vi "BASE_Setting.vi"(8 "error in (no error)":errorcluster) -> (0 "error out":errorcluster)   [LabVIEW 2017]
doc: "this is Hardware setting to set ip address and com port of scanner"
panel:
  in  "System Tab":enum32{"COMMUNICATION SETTING"}(tab)
  in  "HardwareSetting":T1
  in  "Save Button":bool
  in  "Default Button":bool
  in  "Back":bool
  # "BARCODE VERIFICATION SYSTEM REPORTS"
  # "Hardware Setting"
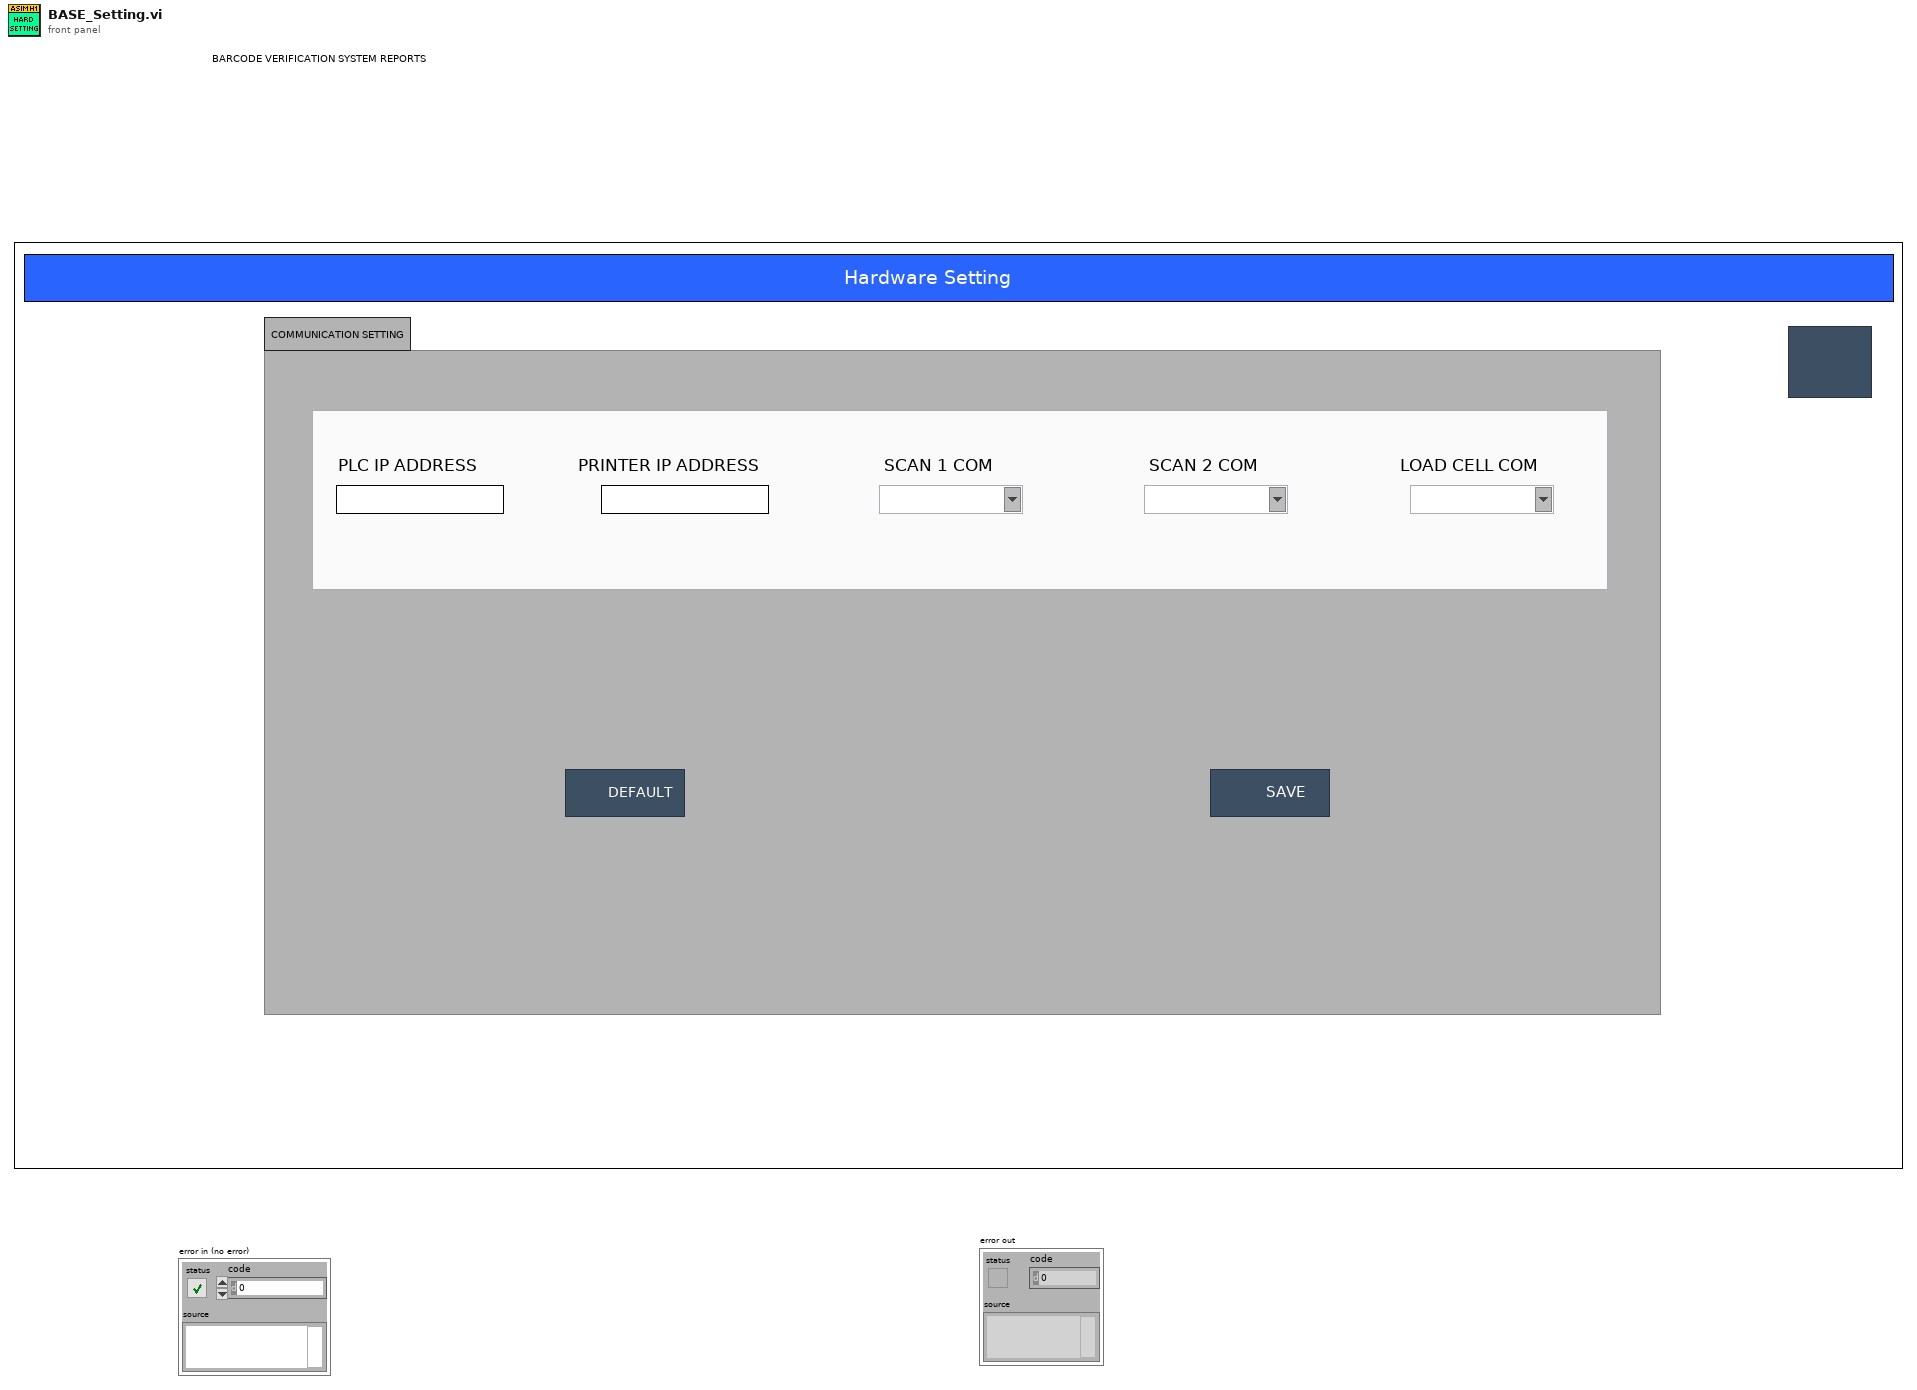
[diagram p1: front panel]
types:
  T1 = cluster{"PLC IP ADDRESS":string, "SCAN 1 COM":refnum<visa-resource-name>, "SCAN 2 COM":refnum<visa-resource-name>, "LOAD CELL COM":refnum<visa-resource-name>, "PRINTER IP ADDRESS":string}
  T2 = enum32{"invalid app kind", "Development System", "Run Time System", "Student Edition", "Embedded LabVIEW", "Evaluation", "Custom"}
  T3 = enum32{"Invalid", "Standard", "Closed", "Hidden", "Minimized", "Maximized"}
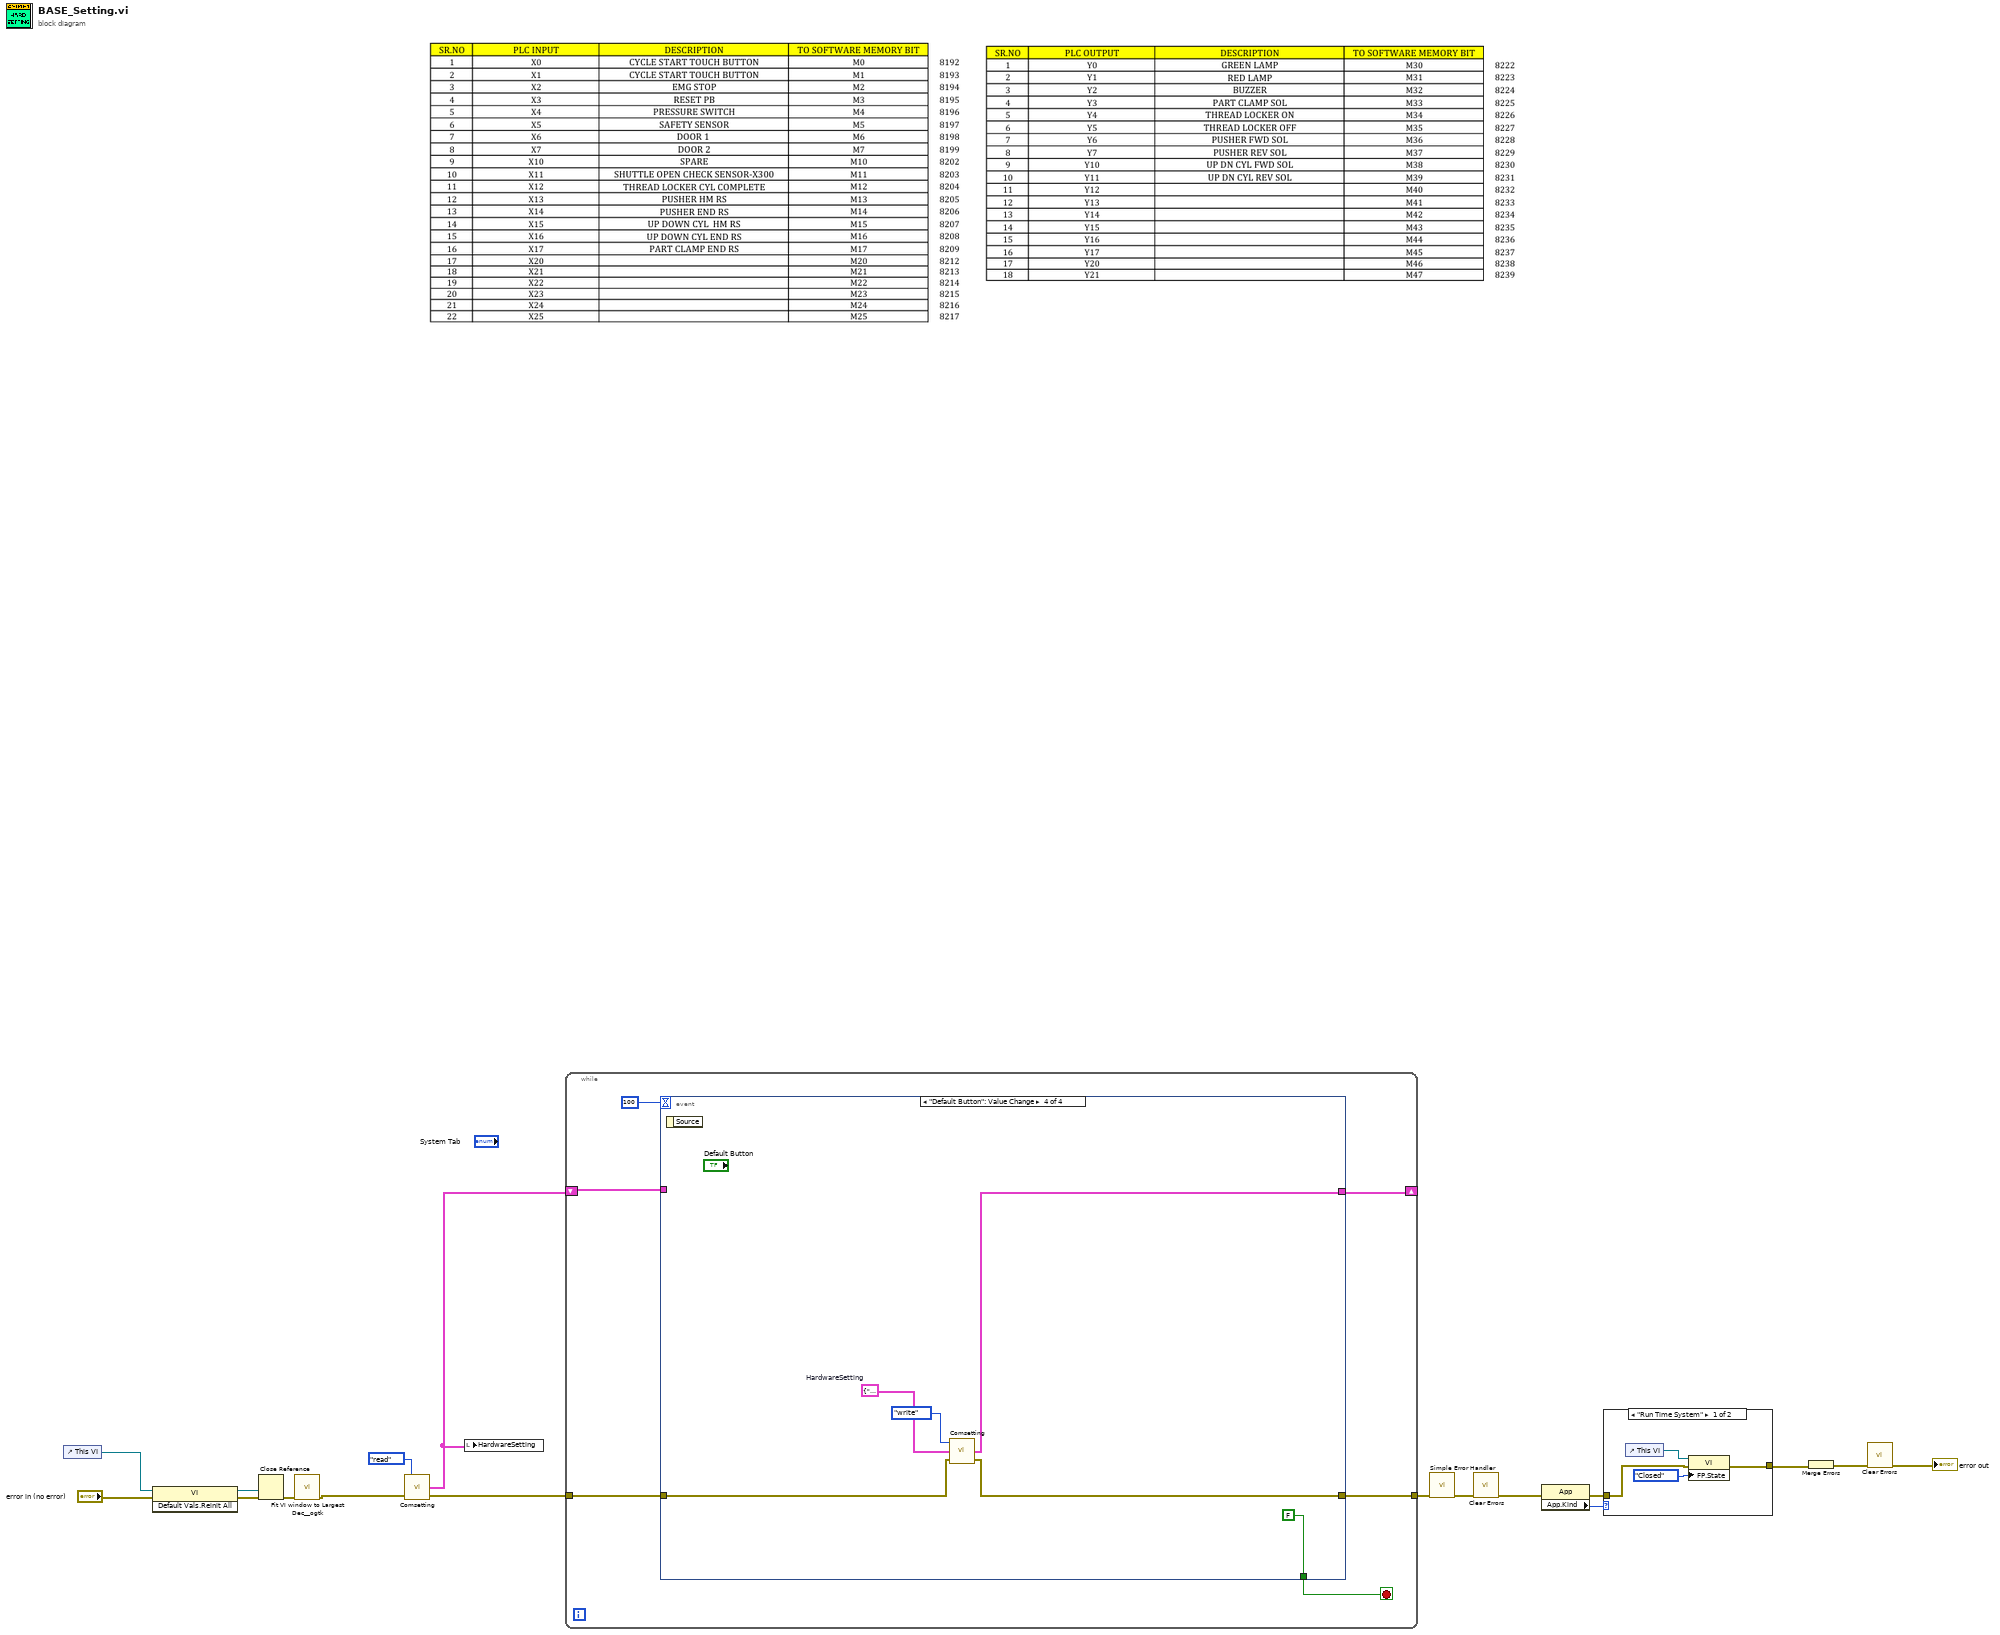
[diagram p0: block diagram]
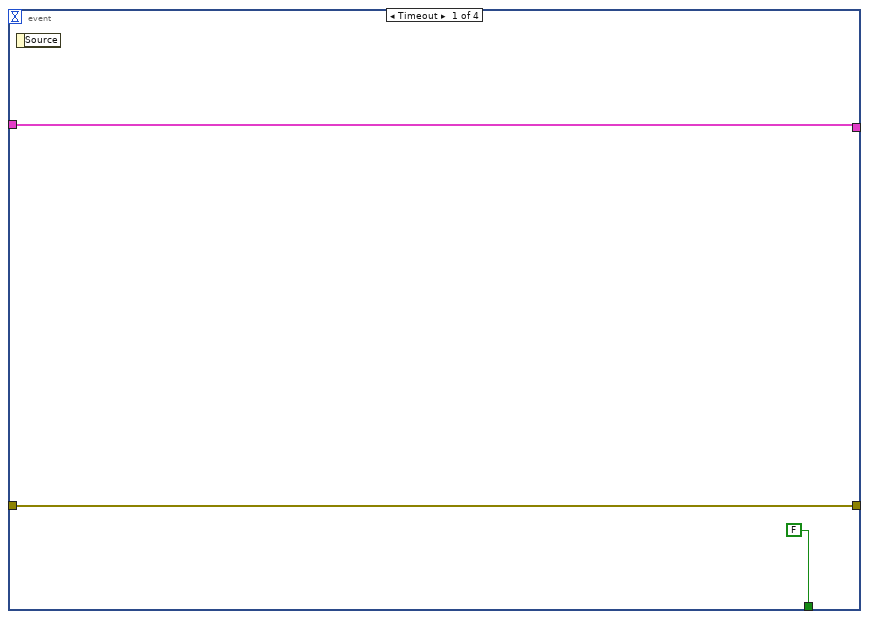
[diagram p2: hidden frame]
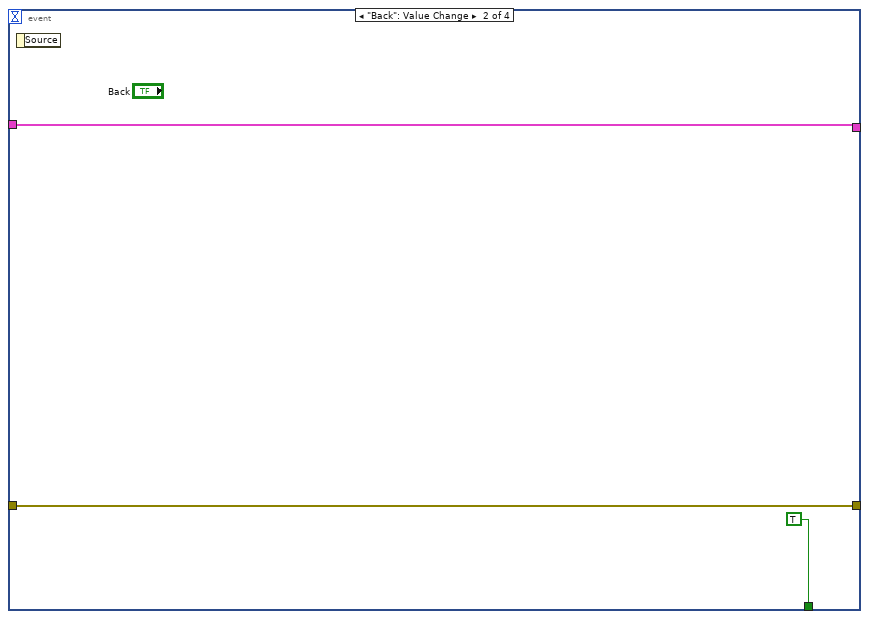
[diagram p3: hidden frame]
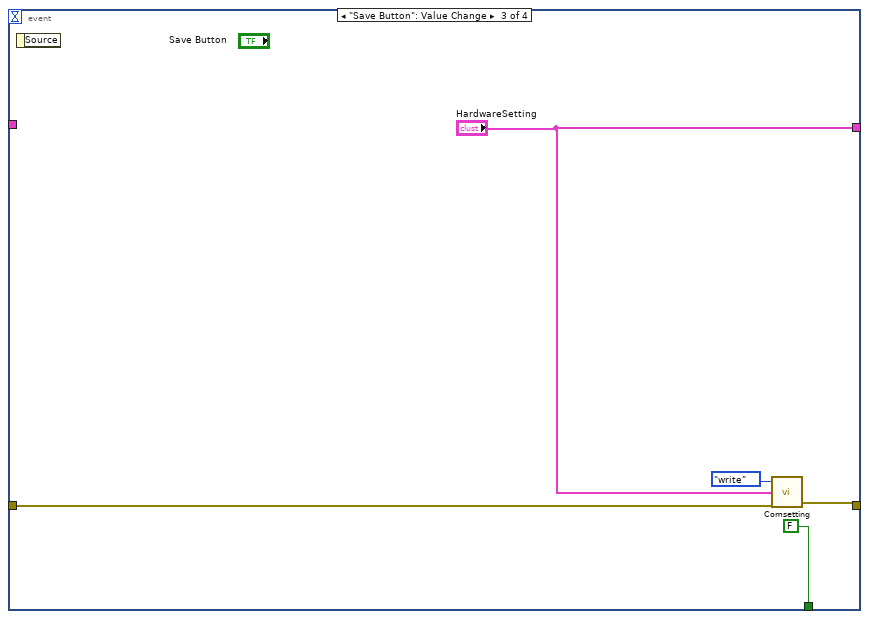
[diagram p4: hidden frame]
diagram:
  n1 = control-ref of="This VI"() -> (w14:refnum<vi>)
  n2 = invoke class="VI" method="Default Vals.Reinit All"(reference=w14, error in="error in (no error)") -> (reference out=w12:refnum<vi>, error out=w11:errorcluster)  [unwired: 1 in, 1 out]
  n3 = Close Reference(reference=w12, error in (no error)=w11) -> (error out=w10:errorcluster)
  n4 = call <userlib>:"Fit VI window to Largest Dec__ogtk.vi"("error in (no error)"=w10) -> ("error out"=w3:errorcluster)  [unwired: 5 in, 1 out]
  n5 = call "Comsetting.vi"("error in"=w3, "Enum"=enum16{"read", "write"}."read") -> ("error our"=w2:errorcluster, "HardwareSetting"=w1:T1)  [unwired: 1 in, 1 out]
  n6 = local write "HardwareSetting"(w1) -> ()
  n7 = while {
    tunnel: [w23] -> w4
    tunnel: w2 -> [w22]
    shift-right: [w21] -> _
    shift-left: w1 -> [w20]
    stop <- w18 stop-if-true
    n8 = event shown="[3] \"Default Button\": Value Change" {
      selector: _ -> [_ _ _ _]
      dyn-events: _ -> [_ _ _ _]
      timeout: 100 -> [_ _ _ _]
      tunnel: [w24 w28 w33 w39] -> w23
      tunnel: w22 -> [w24 w28 w34 w40]
      tunnel: w20 -> [w26 w27 _ _]
      tunnel: [w26 w27 "HardwareSetting" w37] -> w21
      tunnel: [FALSE TRUE FALSE FALSE] -> w18
      event Timeout {
        n9 = event-data() -> ()  [unwired: 1 in, 1 out]
      }
      event "Back": Value Change {
        n10 = event-data() -> ()  [unwired: 1 in, 1 out]
      }
      event "Save Button": Value Change {
        n11 = event-data() -> ()  [unwired: 1 in, 1 out]
        n12 = call "Comsetting.vi"("error in"=w34, "HardwareSetting"="HardwareSetting", "Enum"=enum16{"read", "write"}."write") -> ("error our"=w33:errorcluster)  [unwired: 2 out]
      }
      event "Default Button": Value Change {
        w35 = T1 {"PLC IP ADDRESS"="", "SCAN 1 COM"="", "SCAN 2 COM"="", "LOAD CELL COM"="", "PRINTER IP ADDRESS"=""}  # HardwareSetting
        n13 = event-data() -> ()  [unwired: 1 in, 1 out]
        n14 = call "Comsetting.vi"("error in"=w40, "HardwareSetting"=w35, "Enum"=enum16{"read", "write"}."write") -> ("error our"=w39:errorcluster, "HardwareSetting"=w37:T1)  [unwired: 1 out]
      }
    }
  }
  n15 = call <vilib>:"Simple Error Handler.vi"("error in (no error)"=w4) -> ("error out"=w9:errorcluster)  [unwired: 4 in, 4 out]
  n16 = call <vilib>:"Clear Errors.vi"("error in (no error)"=w9) -> ("error out"=w6:errorcluster)  [unwired: 5 in, 1 out]
  n17 = property class="App"(error in=w6) -> (error out=w7:errorcluster, "App.Kind"=w8:T2)  [unwired: 1 in, 1 out]
  n18 = case shown="\"Run Time System\"" w8 {
    tunnel: w7 -> [w42 w45]
    tunnel: [w41 w45] -> w15
    frame "Run Time System" {
      n19 = control-ref of="This VI"() -> (w44:refnum<vi>)
      n20 = property class="VI"(reference=w44, error in=w42, "FP.State"=T3."Closed" ("Front Panel Window:State")) -> (error out=w41:errorcluster)  [unwired: 1 out]
    }
    frame "Development System", Default {
    }
  }
  n21 = Merge Errors(w15) -> (w16:errorcluster)
  n22 = call <vilib>:"Clear Errors.vi"("error in (no error)"=w16) -> ("error out"=→"error out":errorcluster)  [unwired: 5 in, 1 out]
